vi "GainMeter.vi"() -> ()   [LabVIEW 2015]
uses:
  <vilib>/imath/engines/lvmath2/RunTimeEngine/Managers/WorkSpace/UID Generator.vi
  <vilib>/imath/engines/lvmath2/RunTimeEngine/RunTimeType/NIMS_RunTimeType_From StrictType (excl LVString).vi
  <instcachedir>/0/NIMS_RunTimeType_From StrictType (excl LVString)_EB1C38A9BC5048DA9ABDA8F781E54D21.lvgen/NIMS_RunTimeType_From StrictType (excl LVString)_EB1C38A9BC5048DA9ABDA8F781E54D21_000.vi
  <vilib>/imath/engines/lvmath2/RunTimeEngine/LocalVariableDefStatement/MC_LocalVariableDefStatement_Display.vi
  <vilib>/imath/engines/lvmath2/RunTimeEngine/Managers/SymbolTable/Clear UID.vi
  <vilib>/imath/engines/lvmath2/RunTimeEngine/NodeEndStatement/NIMS_NodeEndStatement_Output.vi
  <instcachedir>/0/NIMS_NodeEndStatement_Output_53EC0D466D134D7ABD903AC30B43404B.lvgen/NIMS_NodeEndStatement_Output_53EC0D466D134D7ABD903AC30B43404B_000.vi
  <vilib>/imath/engines/lvmath2/RunTimeEngine/ErrorHandling/NIMS_Finalize Error.vi
  <vilib>/Analysis/NI_AALPro.lvlib
  <vilib>/imath/engines/lvmath2/RunTimeEngine/Managers/SymbolTable/NIMS_WorkSpace.lvlib
panel:
  out "AC estimate (Vrms)":dbl format="%0.2f"
  out "Numeric":i32
  out "XY Graph":cluster{i32[], "G":dbl[]}(graph)
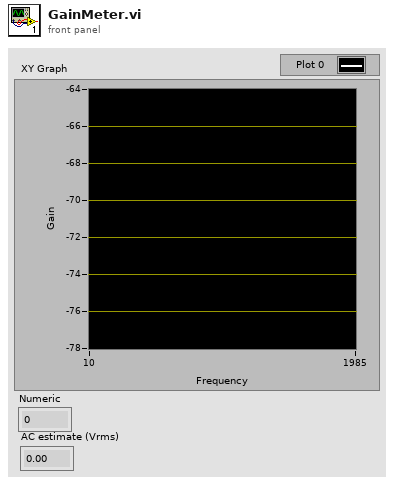
[diagram p1: front panel]
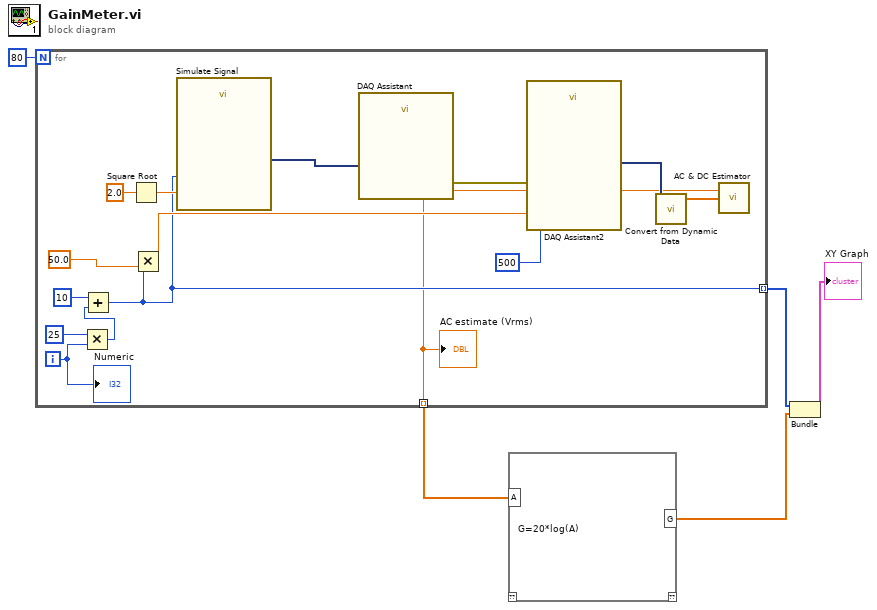
[diagram p0: block diagram]
diagram:
  n1 = for {
    N: 80 -> [_]
    tunnel: [w7] -> w3 mode=indexing
    tunnel: [w6] -> w1 mode=indexing
    i -> [w12]
    n2 = Multiply(x=25, y=w12) -> (x*y=w10:i32)
    n3 = Add(x=10, y=w10) -> (x+y=w7:i32)
    n4 = Square Root(x=2.0) -> (sqrt(x)=w14:dbl)
    n5 = Multiply(x=w7, y=50.0) -> (x*y=w16:dbl)
    n6 = call "Simulate Signal"("Frequency"=w7, "Amplitude"=w14) -> ("Sine"=w8:dynamicdata)  [unwired: 12 in, 1 out]
    n7 = call "DAQ Assistant"("data"=w8) -> ("error out"=w20:errorcluster)  [unwired: 16 in, 2 out]
    n8 = call "DAQ Assistant2"("rate"=w16, "number of samples"=500, "error in"=w20) -> ("data"=w19:dynamicdata)  [unwired: 14 in, 2 out]
    n9 = call "Convert from Dynamic Data"("Dynamic Data Type"=w19) -> ("Array"=w18:dbl[])  [unwired: 3 in]
    n10 = call <vilib>:"AC & DC Estimator.vi"("Signal (V)"=w18) -> ("AC estimate (Vrms)"=w6:dbl)  [unwired: 1 out]
    "AC estimate (Vrms)" <- w6
    "Numeric" <- w12
  }
  n11 = mathscript code="G=20*log(A)"("A"=w1) -> ("G"=w4:cdb[])  [unwired: 1 in, 1 out]
  n12 = Bundle(w3, "G"=w4) -> (→"XY Graph":cluster{i32[], "G":cdb[]})  [unwired: 1 in]
